vi "niScope Cal Adjust Accessory Gain And Offset.vi"(0 "instrument handle":refnum<k15>, 1 "channels":string="0", 2 "posFS":dbl, 3 "gnd":dbl, 4 "negFS":dbl, 5 "error in":errorcluster {"code" format="%.0x"}) -> (14 "instrument handle out":refnum<k15>, 19 "error out":errorcluster={"status"=FALSE, "code"=0, "source"="\n\n"} {"code" format="%.0x"})   [LabVIEW 2013]
doc: "For the NI 5900 differential amplifier, this VI calibrates the gain and offset."
uses:
  niScope_32.dll
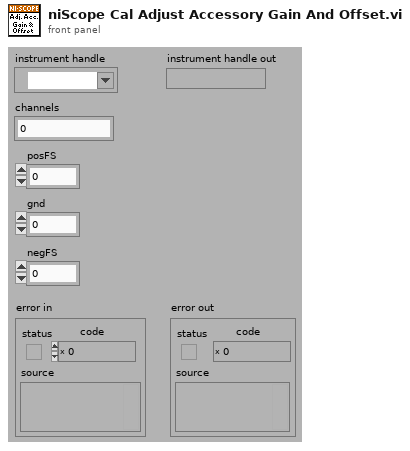
[diagram p1: front panel]
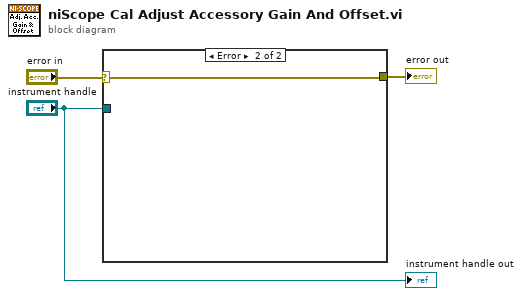
[diagram p0: block diagram]
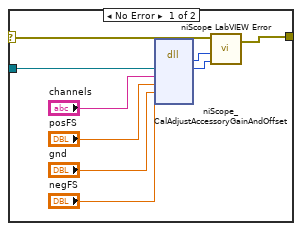
[diagram p2: hidden frame]
diagram:
  n1 = case shown="Error" "error in" {
    selector: "error in" -> [w12 w13]
    tunnel: [w11 w13] -> w2
    tunnel: "instrument handle" -> [w8 _]
    frame No Error {
      n2 = dll-call lib="niScope_*.*" fn="niScope_CalAdjustAccessoryGainAndOffset"("instrumentHandle"=w8, "channelName"="channels", "posFS"="posFS", "gnd"="gnd", "negFS"="negFS") -> (w10:i32, "instrumentHandle"=w9:i32)  [unwired: 7 in, 2 out]
      n3 = call <instrlib>:"niScope LabVIEW Error.vi"("instrument handle"=w9, "niScope error code (0)"=w10, "error in (no error)"=w12) -> ("error out"=w11:errorcluster)  [unwired: 2 in]
    }
    frame Error {
    }
  }
  "error out" <- w2
  "instrument handle out" <- "instrument handle"
